vi "Series I Pump Flow Write SubVI both pumps standalone.vi"(0 "Write to Pump 1?":bool=TRUE, 1 "Write to Pump 2?":bool=TRUE, 3 "Edit or Run/Stop Series IA Pump":string(combo)="Run/Stop", 4 "Stop-Start":bool, 5 "Pump IA Flow Rate (10uL/min)":dbl=3000.0 min=0.0 max=9900.0 step=1.0 format="%0#4_6f", 6 "Stop-Start 2":bool, 7 "error in (no error)":errorcluster, 8 "Pump 1B Flow Rate (10uL/min)":dbl=4000.0 min=0.0 max=9900.0 step=1.0 format="%0#4_6f", 9 "Data Cluster In":T1={"Flom Pump 1 Flow Rate"=0.0, "Script Running"=FALSE, "Unistat Set Temp"=0, "Flom Pump 2 Flow Rate"=0.0, "Flom Pump 1 Running"=FALSE, "Flom Pump 2 Running"=FALSE, "Unistat Running"=FALSE, "Line 1 Flow"=0.0, "Line 2 Flow"=0.0, "Product Temp"=0.0, "Product Flow"=0.0, "HEF Inlet"=0.0, "HEF Outlet"=0.0, "Line 1 Pressure"=0.0, "Line 2 Pressure"=0.0, "Line 3 Pressure"=0.0, "Pump 1 Pressure"=0.0, "Pump 2 Pressure"=0.0, "Number of Steps"=0.0, "Current Step Number"=0.0, "Pump 2 Flow Increment"=0.0, "Step Temp Increment"=0.0, "Step Function Start Time"=0.0, "Pump 2"=FALSE, "Pump 1"=TRUE, "Step Down?"=FALSE, "Number of Cycles"=0.0, "Pump 1 Initial Flow Rate"=0.0, "Pump 2 Initial Flow Rate"=0.0, "Initial Temperature"=0.0, "Step End Time"=0.0, "Pump 1 Current Step Flow"=0.0, "Pump 2 Current Step Flow"=0.0, "Current Step Temp"=0, "Time in each Step"=0.0, "Current Cycle Number"=0.0, "Turn off Temp after Step Flow?"=FALSE, "Internal Temp"=0.0, "Selected Path"=path "", "Excel Row Written"=0, "Counter at constant temp"=0.0, "Temp at Equilibrium"=FALSE, "Temp Equil Counter"=0.0, "Custom Step"=[{"Temp / C"=2, "Time / s"=0, "Flow 2 mL/m"=0.0, "Flow 1 mL/m"=0.0}, {"Temp / C"=2, "Time / s"=20, "Flow 2 mL/m"=0.0, "Flow 1 mL/m"=0.0}, {"Temp / C"=2, "Time / s"=100, "Flow 2 mL/m"=0.0, "Flow 1 mL/m"=0.0}, {"Temp / C"=2, "Time / s"=0, "Flow 2 mL/m"=0.0, "Flow 1 mL/m"=0.0}, {"Temp / C"=2, "Time / s"=90, "Flow 2 mL/m"=0.0, "Flow 1 mL/m"=0.0}, {"Temp / C"=2, "Time / s"=15, "Flow 2 mL/m"=0.0, "Flow 1 mL/m"=0.0}, {"Temp / C"=2, "Time / s"=0, "Flow 2 mL/m"=0.0, "Flow 1 mL/m"=0.0}, {"Temp / C"=2, "Time / s"=75, "Flow 2 mL/m"=0.0, "Flow 1 mL/m"=0.0}, {"Temp / C"=2, "Time / s"=2, "Flow 2 mL/m"=0.0, "Flow 1 mL/m"=0.0}], "Custom Step Number"=0.0, "Current Step t=0?"=FALSE, "Write to File"=FALSE, "Global Initialization Variables"={"Reactor Pressure Hard Upper Limit (bar)"=10.0, "Temp Hard Upper Limit (C)"=80.0, "Temp Hard Lower Limit (C)"=0.0, "Pump Minimum Flow (mL/min)"=0.0, "Pump Maximum Flow (mL/min)"=9.9, "Pump Interval (mL/min)"=0.001, "Temp Interval (C)"=0.1, "Flow Path Volume (mL)"=0.0}, "Error Message"="", "Program Error"=FALSE, "Pump Error"=FALSE, "Hardware Alert"=FALSE, "Comment"="", "Room Temp"=0.0, "VISA Resources"={"Flow VISA"="COM43", "Temp VISA"="COM43", "Flow VISA 1"="COM43", "Flow VISA 2"="COM43", "Flow VISA 3"="COM43", "Pressure VISA"="COM43", "Series IA VISA"="", "Series IB VISA"="", "Flow VISA 4"=""}, "Write Error"=FALSE, "Ports 1-5"=[FALSE, FALSE, FALSE, FALSE, FALSE, FALSE, FALSE, FALSE], "Pump 1 Flow Increment"=0.0, "Send to Product?"=FALSE, "Raman Spectrum Path"=path "", "Raman Spectrum Count"=0.0, "% Yield"=0.0, "Raman File Name"="", "New Spectrum?"=FALSE, "Last Spectrum Collected"=timestamp(0 s since 1904-01-01), "Line 4 Pressure"=0.0, "Series IA Pump Running"=FALSE, "Series IB Pump Running"=FALSE, "Series IA Pump Flow Rate"=0.0, "Series IB Pump Flow Rate"=0.0, "Line 3 Flow"=0.0, "Line 4 Flow"=0.0, "Series IA Pump Pressure"=0.0, "Series IB Pump Pressure"=0.0, "Flow Meter Cal Values"={"Flow Meter 2 Span Flow Rate"=10.0, "Flow Meter 1 Min Counts"=0.0, "Flow Meter 1 Max Counts"=9.9, "Flow Meter 1 Span Flow Rate"=0.01, "Flow Meter 2 Min Counts"=0.1, "Flow Meter 2 Max Counts"=0.0, "Flow Meter 4 Span Flow Rate"=10.0, "Flow Meter 3 Min Counts"=0.0, "Flow Meter 3 Max Counts"=9.9, "Flow Meter 3 Span Flow Rate"=0.01, "Flow Meter 4 Min Counts"=0.1, "Flow Meter 4 Max Counts"=0.0}, "Raman Exp?"=FALSE} {"Global Initialization Variables"."Reactor Pressure Hard Upper Limit (bar)" min=0.0 max=100.0 step=1.0}, 12 "Edit or Run/Stop Series IB Pump":string(combo)="Run/Stop", 13 "Series IA Pump VISA":refnum<visa-resource-name>="COM77", 15 "Series IB Pump VISA":refnum<visa-resource-name>="COM77") -> (20 "Data Cluster Out":T1={"Flom Pump 1 Flow Rate"=0.0, "Script Running"=FALSE, "Unistat Set Temp"=0, "Flom Pump 2 Flow Rate"=0.0, "Flom Pump 1 Running"=FALSE, "Flom Pump 2 Running"=FALSE, "Unistat Running"=FALSE, "Line 1 Flow"=0.0, "Line 2 Flow"=0.0, "Product Temp"=0.0, "Product Flow"=0.0, "HEF Inlet"=0.0, "HEF Outlet"=0.0, "Line 1 Pressure"=0.0, "Line 2 Pressure"=0.0, "Line 3 Pressure"=0.0, "Pump 1 Pressure"=0.0, "Pump 2 Pressure"=0.0, "Number of Steps"=0.0, "Current Step Number"=0.0, "Pump 2 Flow Increment"=0.0, "Step Temp Increment"=0.0, "Step Function Start Time"=0.0, "Pump 2"=FALSE, "Pump 1"=TRUE, "Step Down?"=FALSE, "Number of Cycles"=0.0, "Pump 1 Initial Flow Rate"=0.0, "Pump 2 Initial Flow Rate"=0.0, "Initial Temperature"=0.0, "Step End Time"=0.0, "Pump 1 Current Step Flow"=0.0, "Pump 2 Current Step Flow"=0.0, "Current Step Temp"=0, "Time in each Step"=0.0, "Current Cycle Number"=0.0, "Turn off Temp after Step Flow?"=FALSE, "Internal Temp"=0.0, "Selected Path"=path "", "Excel Row Written"=0, "Counter at constant temp"=0.0, "Temp at Equilibrium"=FALSE, "Temp Equil Counter"=0.0, "Custom Step"=[{"Temp / C"=2, "Time / s"=0, "Flow 2 mL/m"=0.0, "Flow 1 mL/m"=0.0}, {"Temp / C"=2, "Time / s"=20, "Flow 2 mL/m"=0.0, "Flow 1 mL/m"=0.0}, {"Temp / C"=2, "Time / s"=100, "Flow 2 mL/m"=0.0, "Flow 1 mL/m"=0.0}, {"Temp / C"=2, "Time / s"=0, "Flow 2 mL/m"=0.0, "Flow 1 mL/m"=0.0}, {"Temp / C"=2, "Time / s"=90, "Flow 2 mL/m"=0.0, "Flow 1 mL/m"=0.0}, {"Temp / C"=2, "Time / s"=15, "Flow 2 mL/m"=0.0, "Flow 1 mL/m"=0.0}, {"Temp / C"=2, "Time / s"=0, "Flow 2 mL/m"=0.0, "Flow 1 mL/m"=0.0}, {"Temp / C"=2, "Time / s"=75, "Flow 2 mL/m"=0.0, "Flow 1 mL/m"=0.0}, {"Temp / C"=2, "Time / s"=2, "Flow 2 mL/m"=0.0, "Flow 1 mL/m"=0.0}], "Custom Step Number"=0.0, "Current Step t=0?"=FALSE, "Write to File"=FALSE, "Global Initialization Variables"={"Reactor Pressure Hard Upper Limit (bar)"=10.0, "Temp Hard Upper Limit (C)"=80.0, "Temp Hard Lower Limit (C)"=0.0, "Pump Minimum Flow (mL/min)"=0.0, "Pump Maximum Flow (mL/min)"=9.9, "Pump Interval (mL/min)"=0.001, "Temp Interval (C)"=0.1, "Flow Path Volume (mL)"=0.0}, "Error Message"="", "Program Error"=FALSE, "Pump Error"=FALSE, "Hardware Alert"=TRUE, "Comment"="", "Room Temp"=0.0, "VISA Resources"={"Flow VISA"="COM43", "Temp VISA"="COM43", "Flow VISA 1"="COM43", "Flow VISA 2"="COM43", "Flow VISA 3"="COM43", "Pressure VISA"="COM43", "Series IA VISA"="", "Series IB VISA"="", "Flow VISA 4"=""}, "Write Error"=FALSE, "Ports 1-5"=[FALSE, FALSE, FALSE, FALSE, FALSE, FALSE, FALSE, FALSE], "Pump 1 Flow Increment"=0.0, "Send to Product?"=FALSE, "Raman Spectrum Path"=path "", "Raman Spectrum Count"=0.0, "% Yield"=0.0, "Raman File Name"="", "New Spectrum?"=FALSE, "Last Spectrum Collected"=timestamp(0 s since 1904-01-01), "Line 4 Pressure"=0.0, "Series IA Pump Running"=FALSE, "Series IB Pump Running"=FALSE, "Series IA Pump Flow Rate"=0.0, "Series IB Pump Flow Rate"=0.0, "Line 3 Flow"=0.0, "Line 4 Flow"=0.0, "Series IA Pump Pressure"=0.0, "Series IB Pump Pressure"=0.0, "Flow Meter Cal Values"={"Flow Meter 2 Span Flow Rate"=10.0, "Flow Meter 1 Min Counts"=0.0, "Flow Meter 1 Max Counts"=9.9, "Flow Meter 1 Span Flow Rate"=0.01, "Flow Meter 2 Min Counts"=0.1, "Flow Meter 2 Max Counts"=0.0, "Flow Meter 4 Span Flow Rate"=10.0, "Flow Meter 3 Min Counts"=0.0, "Flow Meter 3 Max Counts"=9.9, "Flow Meter 3 Span Flow Rate"=0.01, "Flow Meter 4 Min Counts"=0.1, "Flow Meter 4 Max Counts"=0.0}, "Raman Exp?"=FALSE} {"Global Initialization Variables"."Reactor Pressure Hard Upper Limit (bar)" min=0.0 max=100.0 step=1.0}, 21 "Pump 1A flow rate Out":i32, 25 "Pump 1B flow rate Out":i32, 27 "Error Out":T2)   [LabVIEW 2015]
doc: "Written 12/2010 by Michael Roberto for control and monitoring of Flom high pressure liquid chromatography (HPLC) pumps.\n\nThis VI's purpose is to control the HPLC pumps, in conjunctiton with monitoring pressure and temperature in the reactor, and controlling the temperature via a heating system (yet to be integrated). To do this, the user first chooses the COM port in the VISA resource name box. Then pump number (set up seperately on the pump) is chosen. The user then chooses what kind of interaction they wish to perform with the pump: Continuous Flow, Step Flow, Status, or Reset. Discussion will focus mostly on Continuous and Step Flow commands.\n\nTo execute any command, the EXECUTE button must be pressed, to ensure that the commands are all set and that the pump receives the command only once.\n\nWhen using Continuous Flow, only use the drop down box labeled \"Only for Continuous Flow.\" Using the other boxes or numeric indicators when they're not specifically queried will not cause an error, but it's easier to understand when they're clear or, in the case of step number or time for continuous flow, zero. The flow rate for continuous flow is set seperately from the run/stop command. To edit the flow rate, choose \"edit\" from the drop-down menu and enter a flow rate in the Flow Rate box. Press the EXECUTE button to send the command to the pump. To begin flow, choose \"Start/Stop\" from the drop-down box, and set the switch into the \"Start\" position, and press the EXECUTE button. To stop, switch to Stop and press EXECUTE.\nIn continuous flow, flow rate can be changed while the pump is flowing. Same as before, choose \"edit,\" enter the flow rate, and press EXECUTE.\n\nStep mode is more complicated to run, as flow rates need to be established for each step separately, and the initial flow rate must stipulate how many steps will be executed. I hope to write a VI in the future that, when given a command such as \"20 steps, 0.1 ul/min increments, for 20 minutes,\" will go through and perform these itself, but for now they each have to be performed separately.\n\nGeneric Step Instructions: \nFirst, set up an initial flow rate by choosing such in the drop down menu. It's *important* that you dictate how many steps will be in the program as well. It must be chosen before you hit EXECUTE when setting the initial flow rate.\nSecond, you must define the flow rate and time and step method (linear vs. step) for each step, in the 'configure step' drop down menu. So you would set the step at \"1\", flow rate at the desired flow, and for the desired time length, then press EXECUTE. Then change all those variables again for the 2nd step, and so on. The pump will not recognize commands if you exceed the number of steps dictated in the initial flow rate.\nThird, you run the initial flow rate, by choosing so from the drop down menu and pressing EXECUTE when the switch is in the Start position\nFourth, run the step program.\nAfter the Step Program has finished, the pump will return to the initial flow rate, and will not turn off until you switch to \"Stop\" while in the \"Run initial flow rate\" drop down and hitting EXECUTE."
uses:
  --Controls and TypeDefs--/Control_LDH.ctl
  <vilib>/Instr/_visa.llb/VISA Configure Serial Port (Instr).vi
panel:
  out "String to Send":string
  out "String to Send":string="OK/"
  out "actual bytes read 2":u32=9
  out "Last message received from Pump 1B":string="Pump 2 message, 10:06:19 AM:\nProgram Error: Prohibited command (conflicting operation command)"
  out "Last message received from Pump 1A":string="Pump 1 message, 10:06:19 AM:\nProgram Error: Prohibited command (conflicting operation command)"
  out "actual bytes read":u32=8
  # "SSI Series 1A/1B Pump Control VI.  This VI is a standalone that may be easily converted into a subVI (see comments on block diagram)"
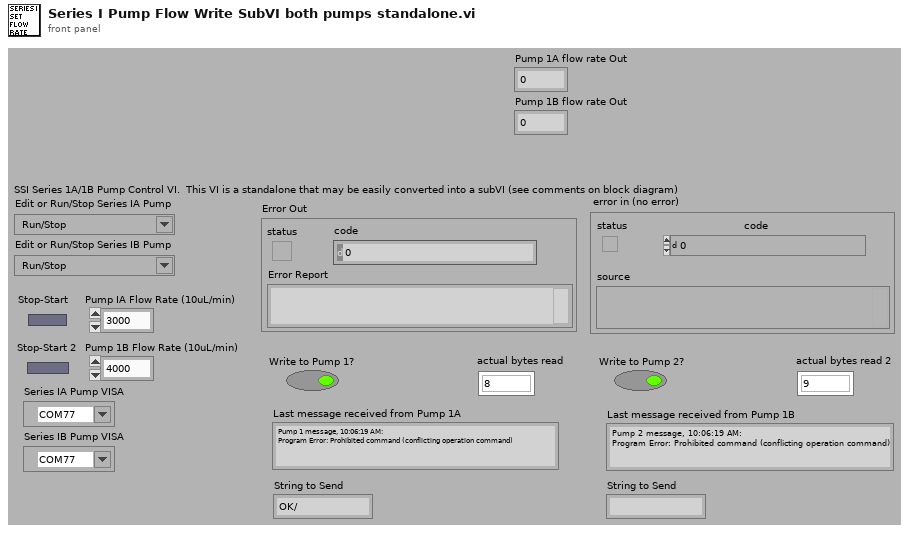
[diagram p1: front panel]
types:
  T1 = typedef "Control_LDH.ctl" = cluster{"Flom Pump 1 Flow Rate":dbl, "Script Running":bool, "Unistat Set Temp":i32, "Flom Pump 2 Flow Rate":dbl, "Flom Pump 1 Running":bool, "Flom Pump 2 Running":bool, "Unistat Running":bool, "Line 1 Flow":dbl, "Line 2 Flow":dbl, "Product Temp":dbl, "Product Flow":dbl, "HEF Inlet":dbl, "HEF Outlet":dbl, "Line 1 Pressure":dbl, "Line 2 Pressure":dbl, "Line 3 Pressure":dbl, "Pump 1 Pressure":dbl, "Pump 2 Pressure":dbl, "Number of Steps":dbl, "Current Step Number":dbl, "Pump 2 Flow Increment":dbl, "Step Temp Increment":dbl, "Step Function Start Time":dbl, "Pump 2":bool, "Pump 1":bool, "Step Down?":bool, "Number of Cycles":dbl, "Pump 1 Initial Flow Rate":dbl, "Pump 2 Initial Flow Rate":dbl, "Initial Temperature":dbl, "Step End Time":dbl, "Pump 1 Current Step Flow":dbl, "Pump 2 Current Step Flow":dbl, "Current Step Temp":i32, "Time in each Step":dbl, "Current Cycle Number":dbl, "Turn off Temp after Step Flow?":bool, "Internal Temp":dbl, "Selected Path":path, "Excel Row Written":i32, "Counter at constant temp":dbl, "Temp at Equilibrium":bool, "Temp Equil Counter":dbl, "Custom Step":cluster{"Temp / C":u16, "Time / s":i32, "Flow 2 mL/m":dbl, "Flow 1 mL/m":dbl}[], "Custom Step Number":dbl, "Current Step t=0?":bool, "Write to File":bool, "Global Initialization Variables":cluster{"Reactor Pressure Hard Upper Limit (bar)":dbl, "Temp Hard Upper Limit (C)":dbl, "Temp Hard Lower Limit (C)":dbl, "Pump Minimum Flow (mL/min)":dbl, "Pump Maximum Flow (mL/min)":dbl, "Pump Interval (mL/min)":dbl, "Temp Interval (C)":dbl, "Flow Path Volume (mL)":dbl}, "Error Message":string, "Program Error":bool, "Pump Error":bool, "Hardware Alert":bool, "Comment":string, "Room Temp":dbl, "VISA Resources":cluster{"Flow VISA":refnum<visa-resource-name>, "Temp VISA":refnum<visa-resource-name>, "Flow VISA 1":refnum<visa-resource-name>, "Flow VISA 2":refnum<visa-resource-name>, "Flow VISA 3":refnum<visa-resource-name>, "Pressure VISA":refnum<visa-resource-name>, "Series IA VISA":refnum<visa-resource-name>, "Series IB VISA":refnum<visa-resource-name>, "Flow VISA 4":refnum<visa-resource-name>}, "Write Error":bool, "Ports 1-5":bool[], "Pump 1 Flow Increment":dbl, "Send to Product?":bool, "Raman Spectrum Path":path, "Raman Spectrum Count":dbl, "% Yield":dbl, "Raman File Name":string, "New Spectrum?":bool, "Last Spectrum Collected":timestamp, "Line 4 Pressure":dbl, "Series IA Pump Running":bool, "Series IB Pump Running":bool, "Series IA Pump Flow Rate":dbl, "Series IB Pump Flow Rate":dbl, "Line 3 Flow":dbl, "Line 4 Flow":dbl, "Series IA Pump Pressure":dbl, "Series IB Pump Pressure":dbl, "Flow Meter Cal Values":cluster{"Flow Meter 2 Span Flow Rate":dbl, "Flow Meter 1 Min Counts":dbl, "Flow Meter 1 Max Counts":dbl, "Flow Meter 1 Span Flow Rate":dbl, "Flow Meter 2 Min Counts":dbl, "Flow Meter 2 Max Counts":dbl, "Flow Meter 4 Span Flow Rate":dbl, "Flow Meter 3 Min Counts":dbl, "Flow Meter 3 Max Counts":dbl, "Flow Meter 3 Span Flow Rate":dbl, "Flow Meter 4 Min Counts":dbl, "Flow Meter 4 Max Counts":dbl}, "Raman Exp?":bool}
  T2 = cluster{"status":bool, "code":i32, "Error Report":string}
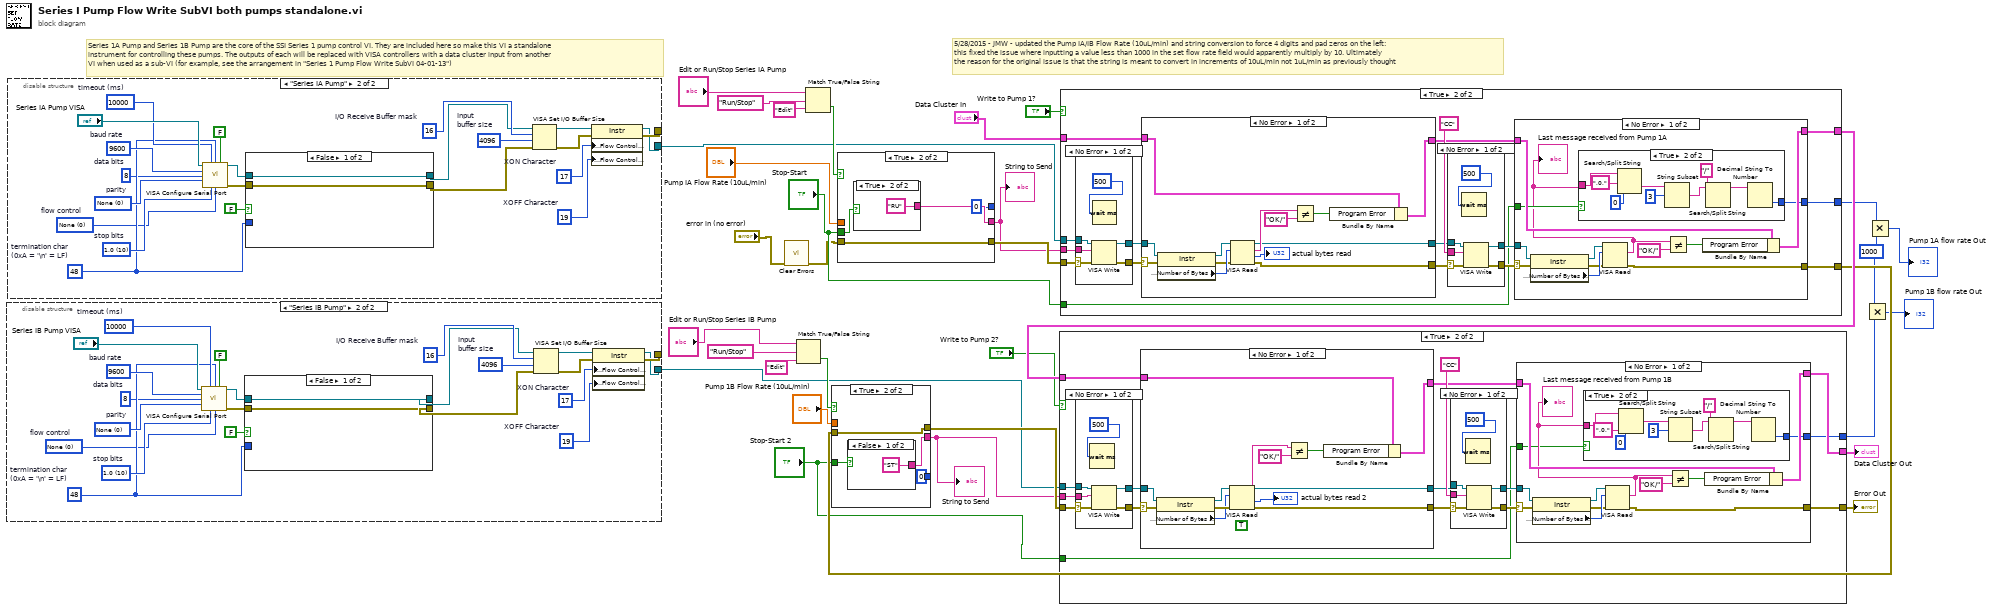
[diagram p0: block diagram]
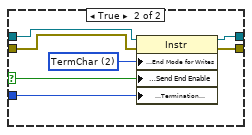
[diagram p3: hidden frame]
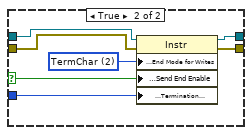
[diagram p5: hidden frame]
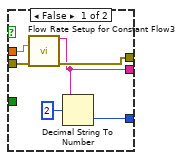
[diagram p6: hidden frame]
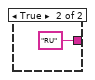
[diagram p7: hidden frame]
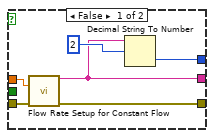
[diagram p8: hidden frame]
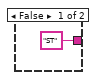
[diagram p9: hidden frame]
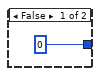
[diagram p11: hidden frame]
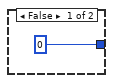
[diagram p17: hidden frame]
diagram:
  w4 = 1000 ("y")
  # "5/28/2015 - JMW - updated the Pump IA/IB Flow Rate (10uL/min) and string conversion to force 4 digits and pad zeros on the left:\nthis fixed the issue where inputting a value less than 1000 in the set flow rate field would apparently multiply by 10. Ultimately\nthe reason for the original issue is that the string is meant to convert in increments of 10uL/min not 1uL/min as previously thought"
  # "Series 1A Pump and Series 1B Pump are the core of the SSI Series 1 pump control VI. They are included here so make this VI a standalone\ninstrument for controlling these pumps. The outputs of each will be replaced with VISA controllers with a data cluster input from another\nVI when used as a sub-VI (for example, see the arrangement in \"Series 1 Pump Flow Write SubVI 04-01-13\")"
  n1 = disable-structure shown="\"Series IB Pump\"" {
    disable-tunnel: [_ w34] -> _
    disable-tunnel: [_ w33] -> w13
    frame condition #0 {
    }
    frame condition #1 (active) {
      w47 = u32 4096  # Input buffer size
      w41 = u8 19  # XOFF Character
      w42 = u8 17  # XON Character
      w50 = u32 10000  # timeout (ms)
      w45 = u8 48  # termination char (0xA = '\n' = LF)
      w44 = u16 0 items=["None"=0, "XON/XOFF"=1, "RTS/CTS"=2, "DTR/DSR"=4]  # flow control
      w51 = u16 10 items=["1.0"=10, "1.5"=15, "2.0"=20]  # stop bits
      w52 = u16 0 items=["None", "Odd", "Even", "Mark", "Space"]  # parity
      w40 = u16 8  # data bits
      w54 = u32 9600  # baud rate
      w48 = u16 16  # I/O Receive Buffer mask
      n2 = call-poly "VISA Configure Serial Port"("VISA resource name"="Series IB Pump VISA", "timeout (10sec)"=w50, "termination char\n(0xA = '\\n' = LF)"=w45, "Enable Termination\nChar (T)"=FALSE ("End read on termination character? 2"), "baud rate (9600)"=w54, "data bits (8)"=w40, "parity (0:none)"=w52, "stop bits (10: 1 bit)"=w51, "flow control (0:none)"=w44) -> ("VISA resource name out"=w37:refnum<visa-resource-name>, "error out"=w39:errorcluster)  [unwired: 1 in, 4 out]
      n3 = case shown="False" FALSE ("End write with termination character? 2") {
        selector: FALSE ("End write with termination character? 2") -> [_ w57]
        tunnel: w37 -> [w55 w63]
        tunnel: w39 -> [w56 w62]
        tunnel: [w55 w61] -> w36
        tunnel: [w56 w60] -> w38
        tunnel: w45 -> [_ w58]
        frame False {
        }
        frame True {
          w59 = u16 2 items=["None", "LastBit", "TermChar", "Break"] ("Serial Settings:Serial End Mode for Writes")
          n4 = property class="Instr"(reference=w63, error in=w62, "Serial Settings:End Mode for Writes"=w59, "Message Based Settings:Send End Enable"=w57, "Message Based Settings:Termination Character"=w58) -> (reference out=w61:refnum<visa-resource-name>, error out=w60:errorcluster)
        }
      }
      n5 = VISA Set I/O Buffer Size(VISA resource name=w36, mask (16)=w48, size (4096)=w47, error in (no error)=w38) -> (VISA resource name out=w35:refnum<visa-resource-name>, error out=w43:errorcluster)
      n6 = property class="Instr"(reference=w35, error in=w43, "Serial Settings:Flow Control XON Character"=w42, "Serial Settings:Flow Control XOFF Character"=w41) -> (reference out=w33:refnum<visa-resource-name>, error out=w34:errorcluster)
    }
  }
  n7 = disable-structure shown="\"Series IA Pump\"" {
    disable-tunnel: [_ w65] -> _
    disable-tunnel: [_ w64] -> w10
    frame condition #0 {
    }
    frame condition #1 (active) {
      w78 = u32 4096  # Input buffer size
      w72 = u8 19  # XOFF Character
      w73 = u8 17  # XON Character
      w81 = u32 10000  # timeout (ms)
      w76 = u8 48  # termination char (0xA = '\n' = LF)
      w75 = u16 0 items=["None"=0, "XON/XOFF"=1, "RTS/CTS"=2, "DTR/DSR"=4]  # flow control
      w82 = u16 10 items=["1.0"=10, "1.5"=15, "2.0"=20]  # stop bits
      w83 = u16 0 items=["None", "Odd", "Even", "Mark", "Space"]  # parity
      w71 = u16 8  # data bits
      w85 = u32 9600  # baud rate
      w79 = u16 16  # I/O Receive Buffer mask
      n8 = call-poly "VISA Configure Serial Port"("VISA resource name"="Series IA Pump VISA", "timeout (10sec)"=w81, "termination char\n(0xA = '\\n' = LF)"=w76, "Enable Termination\nChar (T)"=FALSE ("End read on termination character?"), "baud rate (9600)"=w85, "data bits (8)"=w71, "parity (0:none)"=w83, "stop bits (10: 1 bit)"=w82, "flow control (0:none)"=w75) -> ("VISA resource name out"=w68:refnum<visa-resource-name>, "error out"=w70:errorcluster)  [unwired: 1 in, 4 out]
      n9 = case shown="False" FALSE ("End write with termination character?") {
        selector: FALSE ("End write with termination character?") -> [_ w88]
        tunnel: w68 -> [w86 w94]
        tunnel: w70 -> [w87 w93]
        tunnel: [w86 w92] -> w67
        tunnel: [w87 w91] -> w69
        tunnel: w76 -> [_ w89]
        frame False {
        }
        frame True {
          w90 = u16 2 items=["None", "LastBit", "TermChar", "Break"] ("Serial Settings:Serial End Mode for Writes")
          n10 = property class="Instr"(reference=w94, error in=w93, "Serial Settings:End Mode for Writes"=w90, "Message Based Settings:Send End Enable"=w88, "Message Based Settings:Termination Character"=w89) -> (reference out=w92:refnum<visa-resource-name>, error out=w91:errorcluster)
        }
      }
      n11 = VISA Set I/O Buffer Size(VISA resource name=w67, mask (16)=w79, size (4096)=w78, error in (no error)=w69) -> (VISA resource name out=w66:refnum<visa-resource-name>, error out=w74:errorcluster)
      n12 = property class="Instr"(reference=w66, error in=w74, "Serial Settings:Flow Control XON Character"=w73, "Serial Settings:Flow Control XOFF Character"=w72) -> (reference out=w64:refnum<visa-resource-name>, error out=w65:errorcluster)
    }
  }
  n13 = call <vilib>:"Clear Errors.vi"("error in (no error)"="error in (no error)") -> ("error out"=w1:errorcluster)  [unwired: 5 in, 1 out]
  n14 = Match True/False String(2:"Edit", 3:"Run/Stop", 4:"Edit or Run/Stop Series IB Pump") -> (0:w16:bool)  [unwired: 1 out]
  n15 = Match True/False String(2:"Edit", 3:"Run/Stop", 4:"Edit or Run/Stop Series IA Pump") -> (0:w21:bool)  [unwired: 1 out]
  n16 = case shown="True" w21 {
    tunnel: [w100 w104] -> w28
    tunnel: w1 -> [w99 w104]
    tunnel: "Pump IA Flow Rate (10uL/min)" -> [w98 _]
    tunnel: "Stop-Start" -> [_ w103]
    tunnel: [w96 w102] -> w12
    tunnel: [w95 0] -> _
    frame False {
      n17 = call "Flow Rate Setup for Constant Flow"("flow rate in 10 uL"=w98, "error in (no error)"=w99) -> ("Result"=w96:string, "error out"=w100:errorcluster)  [unwired: 2 in, 10 out]
      n18 = Decimal String To Number(string=w96, offset=2) -> (number=w95:i32)  [unwired: 1 in, 1 out]
    }
    frame True {
      n19 = case shown="True" w103 {
        tunnel: ["ST" "RU"] -> w102
        frame False {
        }
        frame True {
        }
      }
    }
  }
  "String to Send" <- w12
  n20 = case shown="True" "Write to Pump 1?" {
    tunnel: w10 -> [_ w122]
    tunnel: w28 -> [w108 w121]
    tunnel: [w108 w113] -> w15
    tunnel: w12 -> [_ w120]
    tunnel: "Data Cluster In" -> [w107 w119]
    tunnel: [w107 w112] -> w32
    tunnel: "Stop-Start" -> [_ w110]
    tunnel: [_ w109] -> w7
    frame False {
    }
    frame True {
      n21 = case shown="No Error" w121 {
        selector: w121 -> [w176 w180]
        tunnel: [w178 w179] -> w124
        tunnel: [w177 w180] -> w123
        tunnel: w122 -> [w174 w179]
        tunnel: w120 -> [w175 _]
        frame No Error {
          n22 = VISA Write(VISA resource name=w174, write buffer=w175, error in (no error)=w176) -> (VISA resource name out=w178:refnum<visa-resource-name>, error out=w177:errorcluster)  [unwired: 1 out]
          n23 = Wait (ms)(milliseconds to wait=500) -> ()  [unwired: 1 out]
        }
        frame Error {
        }
      }
      n24 = case "Read bytes from port." shown="No Error" w123 {
        selector: w123 -> [w160 w172]
        tunnel: [w166 w172] -> w116
        tunnel: w124 -> [w162 _]
        tunnel: w119 -> [w169 w171]
        tunnel: [w168 w171] -> w114
        tunnel: [w158 _] -> w111
        frame No Error {
          n25 = property class="Instr"(reference=w162, error in=w160) -> (reference out=w161:refnum<visa-resource-name>, error out=w159:errorcluster, "Serial Settings:Number of Bytes at Serial Port"=w163:u32)
          n26 = VISA Read(VISA resource name=w161, byte count=w163, error in (no error)=w159) -> (VISA resource name out=w158:refnum<visa-resource-name>, read buffer=w165:string, return count=→"actual bytes read":u32, error out=w166:errorcluster)
          n27 = Not Equal?(x=w165, y="OK/") -> (x != y?=w164:bool)
          n28 = Bundle By Name(cluster=w169, "Program Error"=w164) -> (w168:T1)
        }
        frame Error {
        }
      }
      n29 = case shown="No Error" w116 {
        selector: w116 -> [w153 w157]
        tunnel: [w155 w156] -> w118
        tunnel: [w154 w157] -> w117
        tunnel: w111 -> [w151 w156]
        tunnel: "CC" -> [w152 _]
        frame No Error {
          n30 = Wait (ms)(milliseconds to wait=500) -> ()  [unwired: 1 out]
          n31 = VISA Write(VISA resource name=w151, write buffer=w152, error in (no error)=w153) -> (VISA resource name out=w155:refnum<visa-resource-name>, error out=w154:errorcluster)  [unwired: 1 out]
        }
        frame Error {
        }
      }
      n32 = case "Read bytes from port." shown="No Error" w117 {
        selector: w117 -> [w129 w149]
        tunnel: [w134 w149] -> w113
        tunnel: w118 -> [w131 _]
        tunnel: w114 -> [w137 w148]
        tunnel: [w136 w148] -> w112
        tunnel: w110 -> [w127 _]
        tunnel: [w125 _] -> w109
        frame No Error {
          n33 = property class="Instr"(reference=w131, error in=w129) -> (reference out=w130:refnum<visa-resource-name>, error out=w128:errorcluster, "Serial Settings:Number of Bytes at Serial Port"=w132:u32)
          n34 = VISA Read(VISA resource name=w130, byte count=w132, error in (no error)=w128) -> (read buffer=w126:string, error out=w134:errorcluster)  [unwired: 2 out]
          "Last message received from Pump 1A" <- w126
          n35 = case shown="True" w127 {
            tunnel: w126 -> [_ w147]
            tunnel: [0 ("y") w139] -> w125
            frame False {
            }
            frame True {
              n36 = Search/Split String(string=w147, search string/char (-)=",0,", offset (0)=0) -> (match + rest of string=w144:string)  [unwired: 2 out]
              n37 = String Subset(string=w144, offset (0)=3) -> (substring=w142:string)  [unwired: 1 in]
              n38 = Search/Split String(string=w142, search string/char (-)="/") -> (substring before match=w140:string)  [unwired: 1 in, 2 out]
              n39 = Decimal String To Number(string=w140) -> (number=w139:i32)  [unwired: 2 in, 1 out]
            }
          }
          n40 = Not Equal?(x=w126, y="OK/") -> (x != y?=w133:bool)
          n41 = Bundle By Name(cluster=w137, "Program Error"=w133) -> (w136:T1)
        }
        frame Error {
        }
      }
    }
  }
  n42 = case shown="True" w16 {
    tunnel: [w186 w190] -> w14
    tunnel: w15 -> [w185 w190]
    tunnel: "Pump 1B Flow Rate (10uL/min)" -> [w184 _]
    tunnel: "Stop-Start 2" -> [_ w189]
    tunnel: [w182 w188] -> w11
    tunnel: [w181 0] -> _
    frame False {
      n43 = call "Flow Rate Setup for Constant Flow3"("flow rate in 10 uL"=w184, "error in (no error)"=w185) -> ("Result"=w182:string, "error out"=w186:errorcluster)  [unwired: 2 in, 10 out]
      n44 = Decimal String To Number(string=w182, offset=2) -> (number=w181:i32)  [unwired: 1 in, 1 out]
    }
    frame True {
      n45 = case shown="False" w189 {
        tunnel: ["ST" "RU"] -> w188
        frame False {
        }
        frame True {
        }
      }
    }
  }
  "String to Send" <- w11
  n46 = case shown="True" "Write to Pump 2?" {
    tunnel: [w193 w198] -> w29
    tunnel: w13 -> [_ w208]
    tunnel: w32 -> [w194 w207]
    tunnel: [w194 w197] -> w31
    tunnel: w11 -> [_ w206]
    tunnel: w14 -> [w193 w205]
    tunnel: "Stop-Start 2" -> [_ w196]
    tunnel: [_ w195] -> w5
    frame False {
    }
    frame True {
      n47 = case shown="No Error" w205 {
        selector: w205 -> [w246 w251]
        tunnel: [w249 w250] -> w210
        tunnel: [w248 w251] -> w209
        tunnel: w208 -> [w247 w250]
        tunnel: w206 -> [w245 _]
        frame No Error {
          n48 = Wait (ms)(milliseconds to wait=500) -> ()  [unwired: 1 out]
          n49 = VISA Write(VISA resource name=w247, write buffer=w245, error in (no error)=w246) -> (VISA resource name out=w249:refnum<visa-resource-name>, error out=w248:errorcluster)  [unwired: 1 out]
        }
        frame Error {
        }
      }
      n50 = case "Read bytes from port." shown="No Error" w209 {
        selector: w209 -> [w258 w265]
        tunnel: [w260 w265] -> w201
        tunnel: w210 -> [w255 _]
        tunnel: w207 -> [w261 _]
        tunnel: [w253 _] -> w200
        tunnel: [w252 _] -> w199
        frame No Error {
          (unwired) TRUE
          n51 = property class="Instr"(reference=w255, error in=w258) -> (reference out=w254:refnum<visa-resource-name>, error out=w257:errorcluster, "Serial Settings:Number of Bytes at Serial Port"=w256:u32)
          n52 = VISA Read(VISA resource name=w254, byte count=w256, error in (no error)=w257) -> (VISA resource name out=w253:refnum<visa-resource-name>, read buffer=w259:string, return count=→"actual bytes read 2":u32, error out=w260:errorcluster)
          n53 = Not Equal?(x=w259, y="OK/") -> (x != y?=w262:bool)
          n54 = Bundle By Name(cluster=w261, "Program Error"=w262) -> (w252:T1)
        }
        frame Error {
        }
      }
      n55 = case shown="No Error" w201 {
        selector: w201 -> [w239 w243]
        tunnel: [w241 w242] -> w204
        tunnel: [w240 w243] -> w203
        tunnel: w200 -> [w237 w242]
        tunnel: "CC" -> [w238 _]
        frame No Error {
          n56 = Wait (ms)(milliseconds to wait=500) -> ()  [unwired: 1 out]
          n57 = VISA Write(VISA resource name=w237, write buffer=w238, error in (no error)=w239) -> (VISA resource name out=w241:refnum<visa-resource-name>, error out=w240:errorcluster)  [unwired: 1 out]
        }
        frame Error {
        }
      }
      n58 = case "Read bytes from port." shown="No Error" w203 {
        selector: w203 -> [w215 w235]
        tunnel: [w220 w235] -> w198
        tunnel: w204 -> [w217 _]
        tunnel: w199 -> [w223 w234]
        tunnel: [w222 w234] -> w197
        tunnel: w196 -> [w212 _]
        tunnel: [w211 _] -> w195
        frame No Error {
          n59 = property class="Instr"(reference=w217, error in=w215) -> (reference out=w216:refnum<visa-resource-name>, error out=w214:errorcluster, "Serial Settings:Number of Bytes at Serial Port"=w218:u32)
          n60 = VISA Read(VISA resource name=w216, byte count=w218, error in (no error)=w214) -> (read buffer=w213:string, error out=w220:errorcluster)  [unwired: 2 out]
          "Last message received from Pump 1B" <- w213
          n61 = case shown="True" w212 {
            tunnel: w213 -> [_ w233]
            tunnel: [0 ("y") w225] -> w211
            frame False {
            }
            frame True {
              n62 = Search/Split String(string=w233, search string/char (-)=",0,", offset (0)=0) -> (match + rest of string=w226:string)  [unwired: 2 out]
              n63 = String Subset(string=w226, offset (0)=3) -> (substring=w228:string)  [unwired: 1 in]
              n64 = Search/Split String(string=w228, search string/char (-)="/") -> (substring before match=w230:string)  [unwired: 1 in, 2 out]
              n65 = Decimal String To Number(string=w230) -> (number=w225:i32)  [unwired: 2 in, 1 out]
            }
          }
          n66 = Not Equal?(x=w213, y="OK/") -> (x != y?=w219:bool)
          n67 = Bundle By Name(cluster=w223, "Program Error"=w219) -> (w222:T1)
        }
        frame Error {
        }
      }
    }
  }
  "Error Out" <- w29
  "Data Cluster Out" <- w31
  n68 = Multiply(x=w4, y=w5) -> (x*y=→"Pump 1B flow rate Out":i32)
  n69 = Multiply(x=w7, y=w4) -> (x*y=→"Pump 1A flow rate Out":i32)
